vi "Word Check.vi"(9 "Any":string, 10 "Word_Ref":refnum<vi>, 11 "Word":T1) -> (3 "IsOk":bool)   [LabVIEW 2015]
uses:
  TypeDef/Word.ctl
  TypeDef/Color.ctl
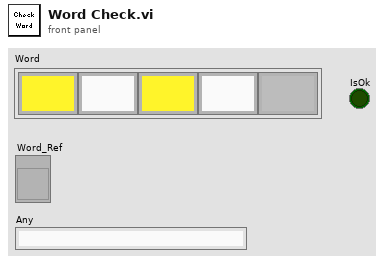
[diagram p1: front panel]
types:
  T1 = typedef "Word.ctl" = cluster{"1":string, "2":string, "3":string, "4":string, "5":string}
  T2 = typedef "Color.ctl" = u32
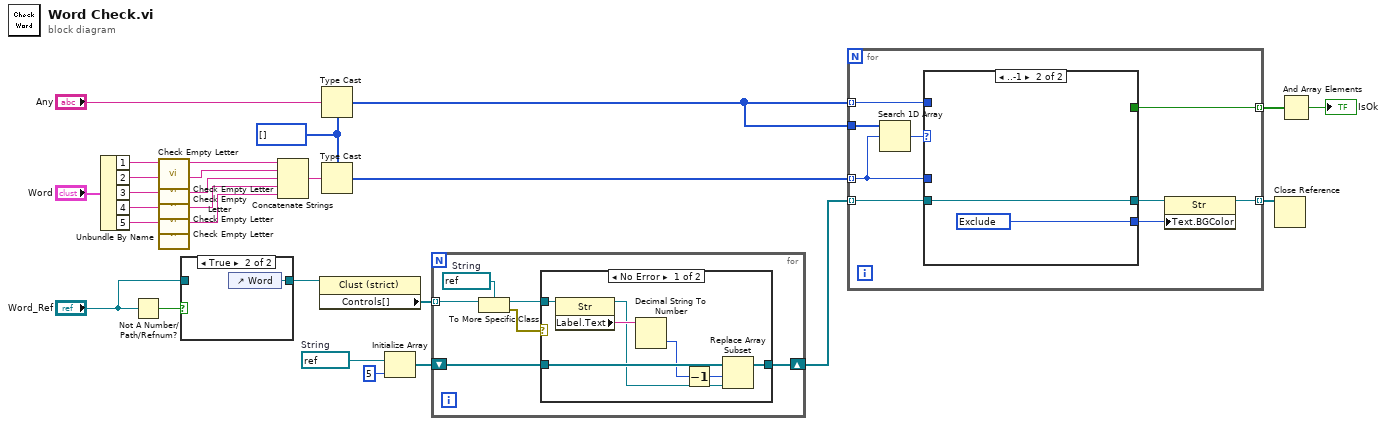
[diagram p0: block diagram]
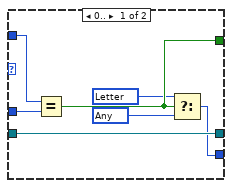
[diagram p4: hidden frame]
diagram:
  w17 = u8[] []
  w20 = refnum<vi> refnum  # String
  n1 = Unbundle By Name("Word") -> ("1"=w12:string, "2"=w11:string, "3"=w10:string, "4"=w9:string, "5"=w8:string)
  n2 = Not A Number/Path/Refnum?(number/path/refnum="Word_Ref") -> (NaN/Path/Refnum?=w27:bool)
  n3 = call "Check Empty Letter.vi"("Letter in"=w12) -> ("Letter Out"=w7:string)  [unwired: 10 in]
  n4 = call "Check Empty Letter.vi"("Letter in"=w11) -> ("Letter Out"=w6:string)  [unwired: 10 in]
  n5 = call "Check Empty Letter.vi"("Letter in"=w10) -> ("Letter Out"=w5:string)  [unwired: 10 in]
  n6 = call "Check Empty Letter.vi"("Letter in"=w9) -> ("Letter Out"=w4:string)  [unwired: 10 in]
  n7 = call "Check Empty Letter.vi"("Letter in"=w8) -> ("Letter Out"=w3:string)  [unwired: 10 in]
  n8 = case shown="True" w27 {
    tunnel: "Word_Ref" -> [w28 _]
    tunnel: [w28 w29] -> w24
    frame False {
    }
    frame True {
      n9 = control-ref of="Word"() -> (w29:refnum<vi>)
    }
  }
  n10 = Concatenate Strings(w7, w6, w5, w4, w3) -> (w19:string)
  n11 = property class="Clust (strict)"(reference=w24) -> ("Controls[]"=w23:refnum<vi>[])  [unwired: 1 in, 2 out]
  n12 = Type Cast(type=w17, x="Any") -> (*(type *) &x=w15:u8[])
  n13 = Type Cast(type=w17, x=w19) -> (*(type *) &x=w16:u8[])
  n14 = Initialize Array(w20, 5 ("dimension size")) -> (w21:refnum<vi>[])
  n15 = for {
    tunnel: w23 -> [w33] mode=indexing
    shift-right: [w34] -> w14
    shift-left: w21 -> [w35]
    w31 = refnum<vi> refnum  # String
    n16 = To More Specific Class(target class=w31, reference=w33) -> (specific class reference=w32:refnum<vi>, error out=w30:errorcluster)  [unwired: 1 in]
    n17 = case shown="No Error" w30 {
      tunnel: w35 -> [w41 w43]
      tunnel: [w40 w43] -> w34
      tunnel: w32 -> [w38 _]
      frame No Error {
        n18 = property class="Str"(reference=w38) -> (reference out=w37:refnum<vi>, "Label.Text"=w42:string)  [unwired: 1 in, 1 out]
        n19 = Decimal String To Number(string=w42) -> (number=w39:i32)  [unwired: 2 in, 1 out]
        n20 = Decrement(x=w39) -> (x-1=w36:i32)
        n21 = Replace Array Subset(array=w41, new element=w37, index=w36) -> (w40:refnum<vi>[])
      }
      frame Error {
      }
    }
  }
  n22 = for {
    tunnel: w16 -> [w48] mode=indexing
    tunnel: w15 -> [w49] mode=indexing
    tunnel: w15 -> [w52]
    tunnel: w14 -> [w50] mode=indexing
    tunnel: [w46] -> w13 mode=indexing
    tunnel: [w44] -> w2 mode=indexing
    n23 = Search 1D Array(1D array=w52, element=w48) -> (index of element=w51:i32)  [unwired: 1 in]
    n24 = case shown="..-1" w51 {
      tunnel: w50 -> [w59 w61]
      tunnel: [w59 w61] -> w47
      tunnel: w49 -> [w58 _]
      tunnel: w48 -> [w57 _]
      tunnel: [w56 w60] -> w45
      tunnel: [w55 _] -> w44
      frame 0.. {
        w53 = T2 16448250 items=["Free"=9567230, "Letter"=16774186, "Any"=16448250, "Exclude"=12369084] ("Color")
        w54 = T2 16774186 items=["Free"=9567230, "Letter"=16774186, "Any"=16448250, "Exclude"=12369084] ("Color")
        n25 = Equal?(x=w58, y=w57) -> (x = y?=w55:bool)
        n26 = Select(t=w54, s=w55, f=w53) -> (s? t:f=w56:T2)
      }
      frame ..-1 {
        w60 = T2 12369084 items=["Free"=9567230, "Letter"=16774186, "Any"=16448250, "Exclude"=12369084] ("Color")
      }
    }
    n27 = property class="Str"(reference=w47, "Text.BGColor"=w45) -> (reference out=w46:refnum<vi>)  [unwired: 1 in, 1 out]
  }
  n28 = Close Reference(reference=w13) -> ()  [unwired: 1 in, 1 out]
  n29 = And Array Elements(Boolean array=w2) -> (logical AND=→"IsOk":bool)
